vi "Build queue.vi"(8 "Scan settings array":T1[](array[typedef]) {"J-t Illumination conditions" items=["Light only", "Dark only", "Light then dark", "Dark then light"]; "No. of scan rate steps" min=1.0 step=1.0; "Illumination conditions" items=["Light only", "Dark only", "Light then dark", "Dark then light", "Light then dark then light", "Dark then light then dark"]; "Time Constant (s)" items=["0.003", "0.01", "0.03", "0.1", "0.3", "1", "3", "10", "30", "100"]; "Only repeat for best pixel" items=["only for best pixel", "for best 2 pixels", "for best 3 pixels", "for best 4 pixels", "for best 5 pixels", "for best 6 pixels", "for best 7 pixels", "for all pixels"]; "No. of repeat scans" min=1.0 step=1.0; "EQE best pixel only" items=["only the best pixel", "the best 2 pixel", "the best 3 pixel", "the best 4 pixel", "the best 5 pixel", "the best 6 pixel", "the best 7 pixel", "all pixels"]; "P dep best pixel only" items=["only the best pixel", "the best 2 pixels", "the best 3 pixels", "the best 4 pixels", "the best 5 pixels", "the best 6 pixels", "the best 7 pixels", "all pixels"]; "Max power best pixel only" items=["only the best pixel", "the best 2 pixels", "the best 3 pixels", "the best 4 pixels", "the best 5 pixels", "the best 6 pixels", "the best 7 pixels", "all pixels"]; "J-t best pixel only" items=["only the best pixel", "the best 2 pixels", "the best 3 pixels", "the best 4 pixels", "the best 5 pixels", "the best 6 pixels", "the best 7 pixels", "all pixels"]; "Integration time" items=["Fast", "Normal", "High Accuracy"]; "Stabilisation mode" items=["V", "I"]; "Measurement delay (ms)" min=10.0}, 11 "Cell Settings Array":T4(array[cluster])=[{"Cell Position"=1, "Cell Label"="", "Pixel to measure"=0, "Area (cm^2)"=0.126, "Variable"="", "Variable value"="", "Scan settings in queue"=0}, {"Cell Position"=2, "Cell Label"="", "Pixel to measure"=0, "Area (cm^2)"=0.126, "Variable"="", "Variable value"="", "Scan settings in queue"=0}, {"Cell Position"=3, "Cell Label"="", "Pixel to measure"=0, "Area (cm^2)"=0.126, "Variable"="", "Variable value"="", "Scan settings in queue"=0}, {"Cell Position"=4, "Cell Label"="", "Pixel to measure"=0, "Area (cm^2)"=0.126, "Variable"="", "Variable value"="", "Scan settings in queue"=0}, {"Cell Position"=5, "Cell Label"="", "Pixel to measure"=0, "Area (cm^2)"=0.126, "Variable"="", "Variable value"="", "Scan settings in queue"=0}, {"Cell Position"=6, "Cell Label"="", "Pixel to measure"=0, "Area (cm^2)"=0.126, "Variable"="", "Variable value"="", "Scan settings in queue"=0}, {"Cell Position"=7, "Cell Label"="", "Pixel to measure"=0, "Area (cm^2)"=0.126, "Variable"="", "Variable value"="", "Scan settings in queue"=0}, {"Cell Position"=8, "Cell Label"="", "Pixel to measure"=0, "Area (cm^2)"=0.126, "Variable"="", "Variable value"="", "Scan settings in queue"=0}, {"Cell Position"=9, "Cell Label"="", "Pixel to measure"=0, "Area (cm^2)"=0.126, "Variable"="", "Variable value"="", "Scan settings in queue"=0}, {"Cell Position"=10, "Cell Label"="", "Pixel to measure"=0, "Area (cm^2)"=0.126, "Variable"="", "Variable value"="", "Scan settings in queue"=0}, {"Cell Position"=11, "Cell Label"="", "Pixel to measure"=0, "Area (cm^2)"=0.126, "Variable"="", "Variable value"="", "Scan settings in queue"=0}, {"Cell Position"=12, "Cell Label"="", "Pixel to measure"=0, "Area (cm^2)"=0.126, "Variable"="", "Variable value"="", "Scan settings in queue"=0}, {"Cell Position"=13, "Cell Label"="", "Pixel to measure"=0, "Area (cm^2)"=0.126, "Variable"="", "Variable value"="", "Scan settings in queue"=0}, {"Cell Position"=14, "Cell Label"="", "Pixel to measure"=0, "Area (cm^2)"=0.126, "Variable"="", "Variable value"="", "Scan settings in queue"=0}, {"Cell Position"=15, "Cell Label"="", "Pixel to measure"=0, "Area (cm^2)"=0.126, "Variable"="", "Variable value"="", "Scan settings in queue"=0}, {"Cell Position"=16, "Cell Label"="", "Pixel to measure"=0, "Area (cm^2)"=0.126, "Variable"="", "Variable value"="", "Scan settings in queue"=0}] {"Pixel to measure" items=["All", "1", "2", "3", "4", "5", "6", "7", "8"]}) -> (3 "Measurement queue":T3(array[cluster]) {"Pixel to measure" items=["All", "1", "2", "3", "4", "5", "6", "7", "8"]})   [LabVIEW 2011]
uses:
  TypeDefs/Scan settings.ctl
  TypeDefs/Settings Boolean.ctl
panel:
  out "Max power best pixel only":u16
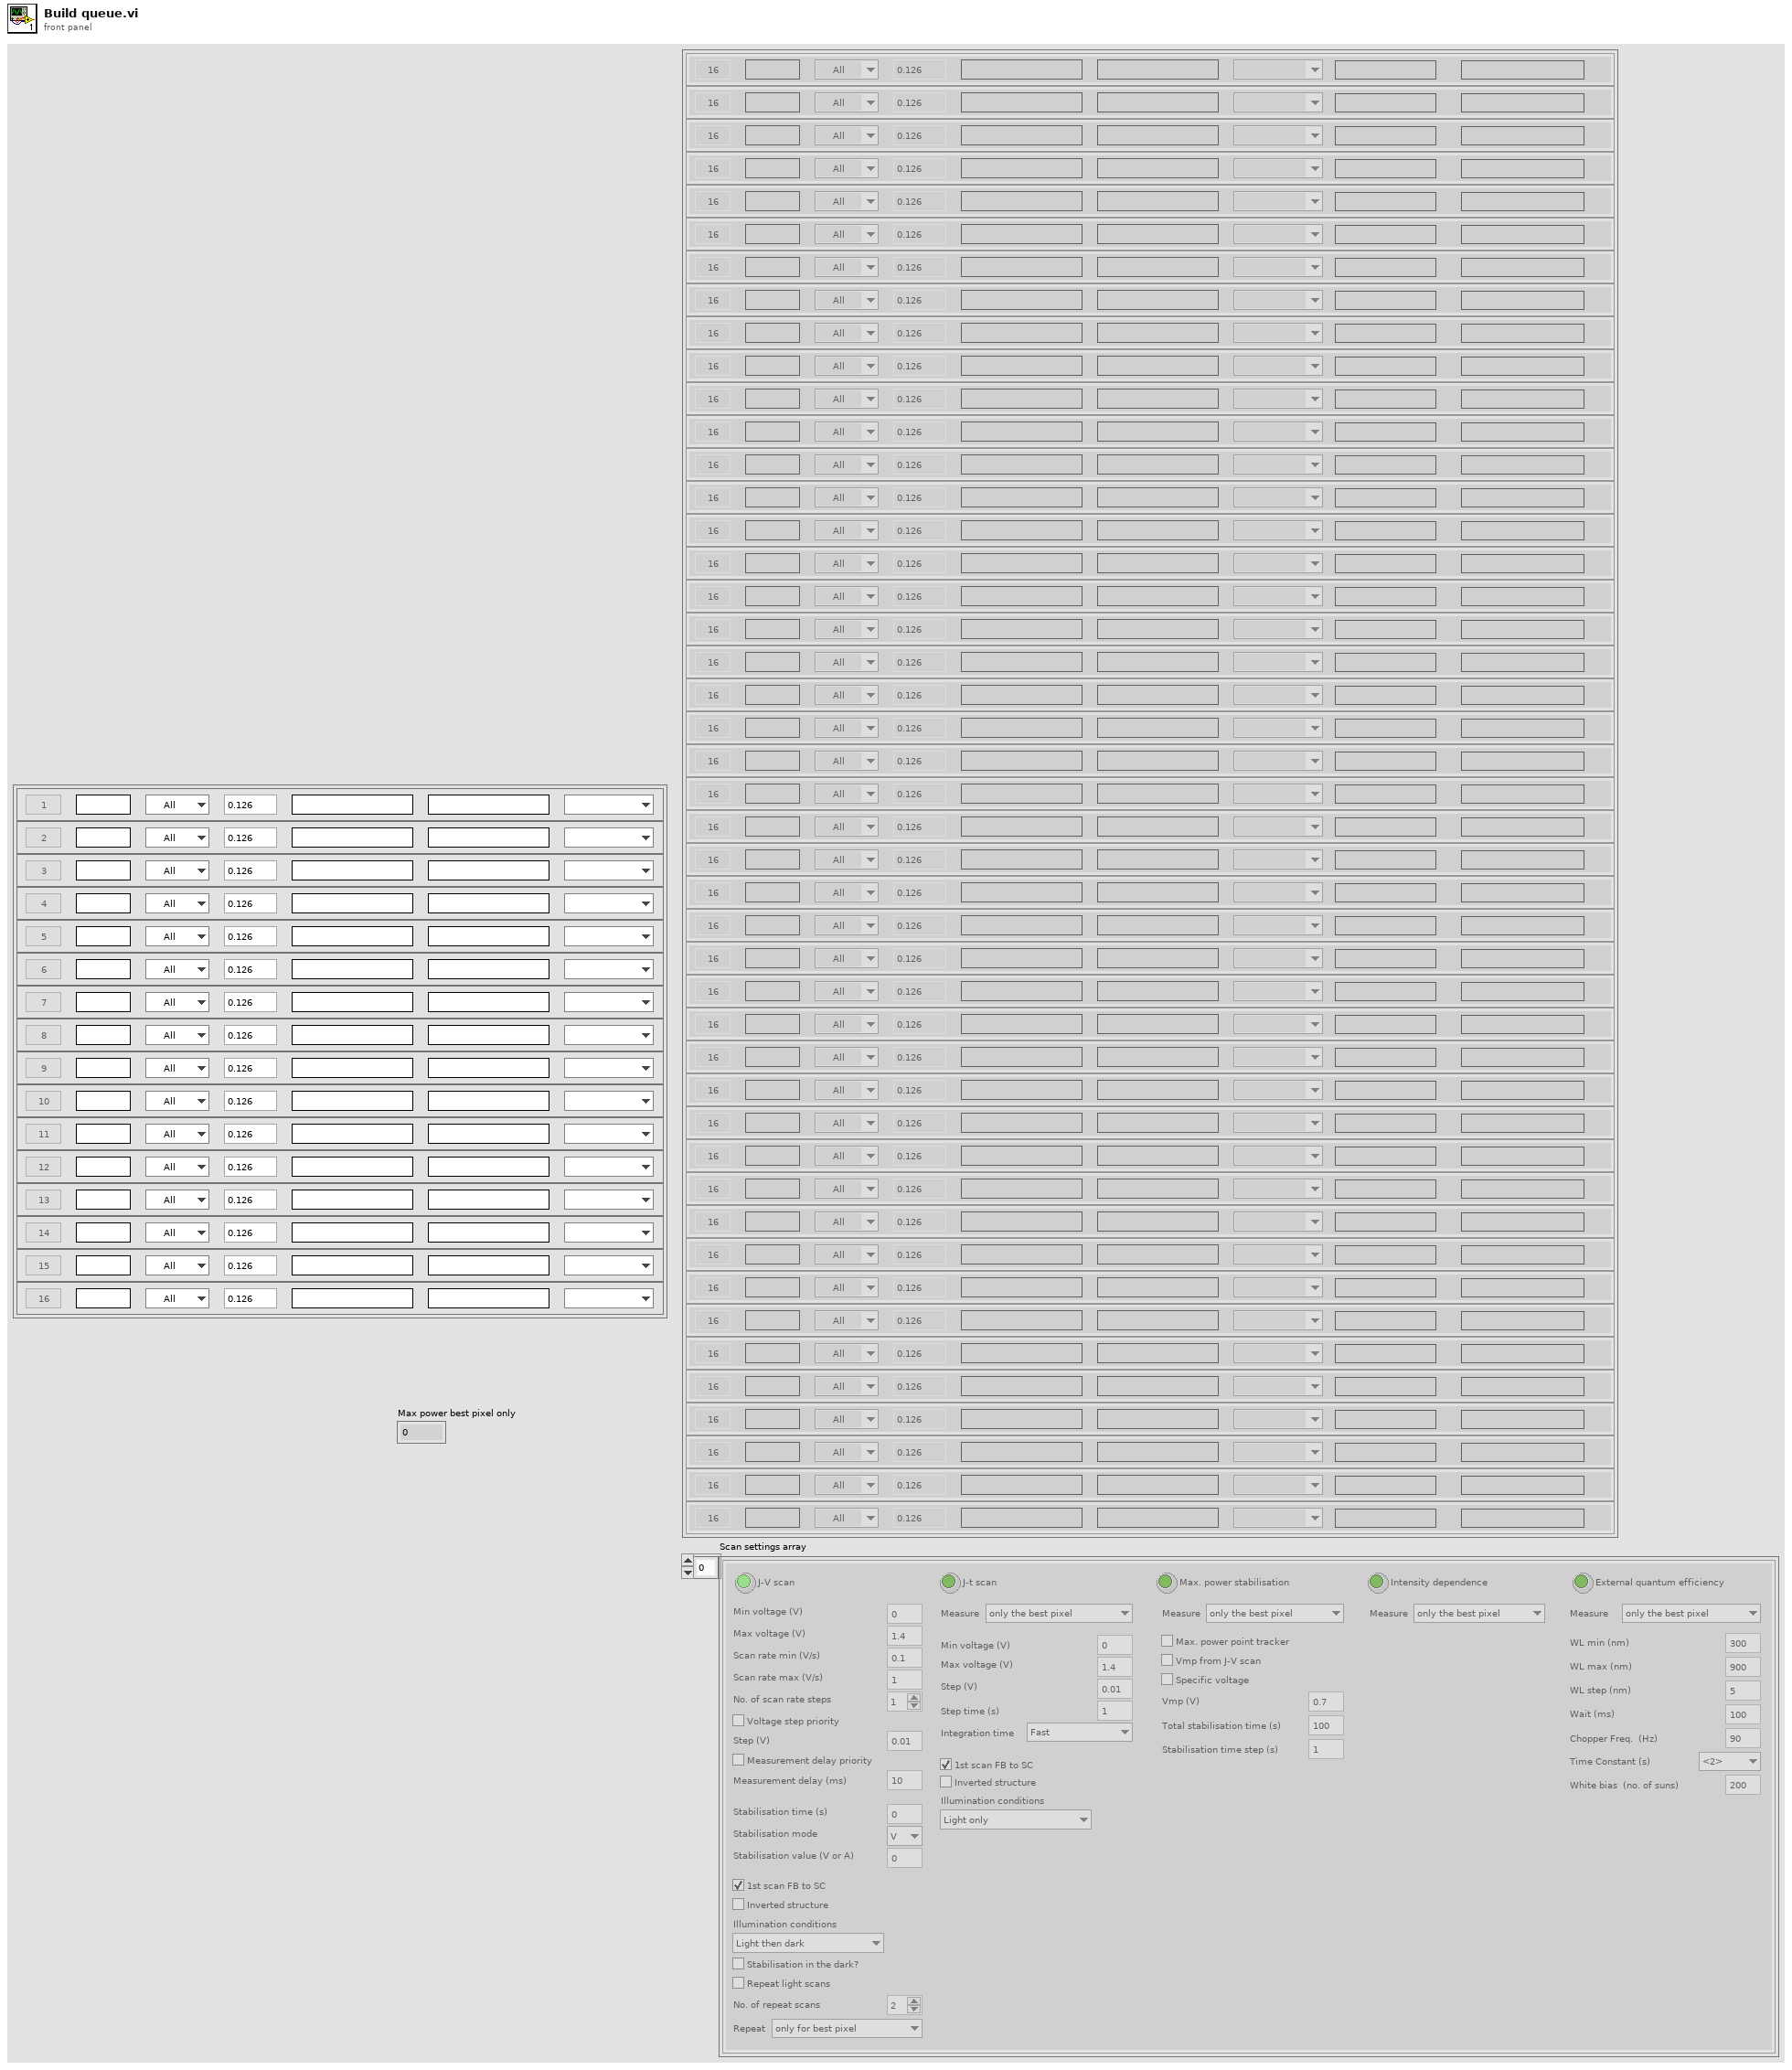
[diagram p1: front panel]
types:
  T1 = typedef "Scan settings.ctl" = cluster{"J-V scan":T2, "J-t scan":bool, "Min voltage (V)":dbl, "Max voltage (V)":dbl, "Step (V)":dbl, "Measurement delay (ms)":dbl, "1st scan FB-SC":bool, "Inverted structure":bool, "Stabilisation time (s)":dbl, "Stabilisation mode":u16, "Stabilisation value (V or A) ":dbl, "Step time (s)":dbl, "Integration time":u16, "Repeat light scans":bool, "Stabilisation in the dark?":bool, "J-t Min (V)":dbl, "J-t Max (V)":dbl, "J-t Step (V)":dbl, "Max. power stabilisation":bool, "J-t 1st scan FB-SC":bool, "J-t Inverted structure":bool, "Max power tracking":bool, "Vmp (V)":dbl, "Total stabilisation time (s)":dbl, "J-t best pixel only":u16, "Max power best pixel only":u16, "Vmp from J-V scan":bool, "Intensity dependence":bool, "P dep best pixel only":u16, "External quantum efficiency":bool, "EQE best pixel only":u16, "WL min (nm)":dbl, "WL max (nm)":dbl, "WL step (nm)":dbl, "Wait (ms)":dbl, "No. of repeat scans":dbl, "Only repeat for best pixel":u16, "Chopper Freq.  (Hz)":dbl, "Time Constant (s)":dbl, "Stabilisation time step (s)":dbl, "Illumination conditions":u16, "Scan rate min (V/s)":dbl, "Scan rate max (V/s)":dbl, "No. of scan rate steps":dbl, "Scan rate voltage step priority":bool, "Scan rate measurement delay priority":bool, "J-t Illumination conditions":u16, "White bias  (no. of suns)":dbl, "Max P stab. Specific voltage":bool}
  T2 = typedef "Settings Boolean.ctl" = bool
  T3 = cluster{"Cell Position":i32, "Cell Label":string, "Pixel to measure":u16, "Area (cm^2)":dbl, "Variable":string, "Variable value":string, "Scan settings in queue":u16, "Light or dark":string, "Measurement type":string}[]
  T4 = cluster{"Cell Position":i32, "Cell Label":string, "Pixel to measure":u16, "Area (cm^2)":dbl, "Variable":string, "Variable value":string, "Scan settings in queue":u16}[]
  T5 = cluster{"Cell Position":i32, "Cell Label":string, "Pixel to measure":u16, "Area (cm^2)":dbl, "Variable":string, "Variable value":string, "Scan settings in queue":u16}
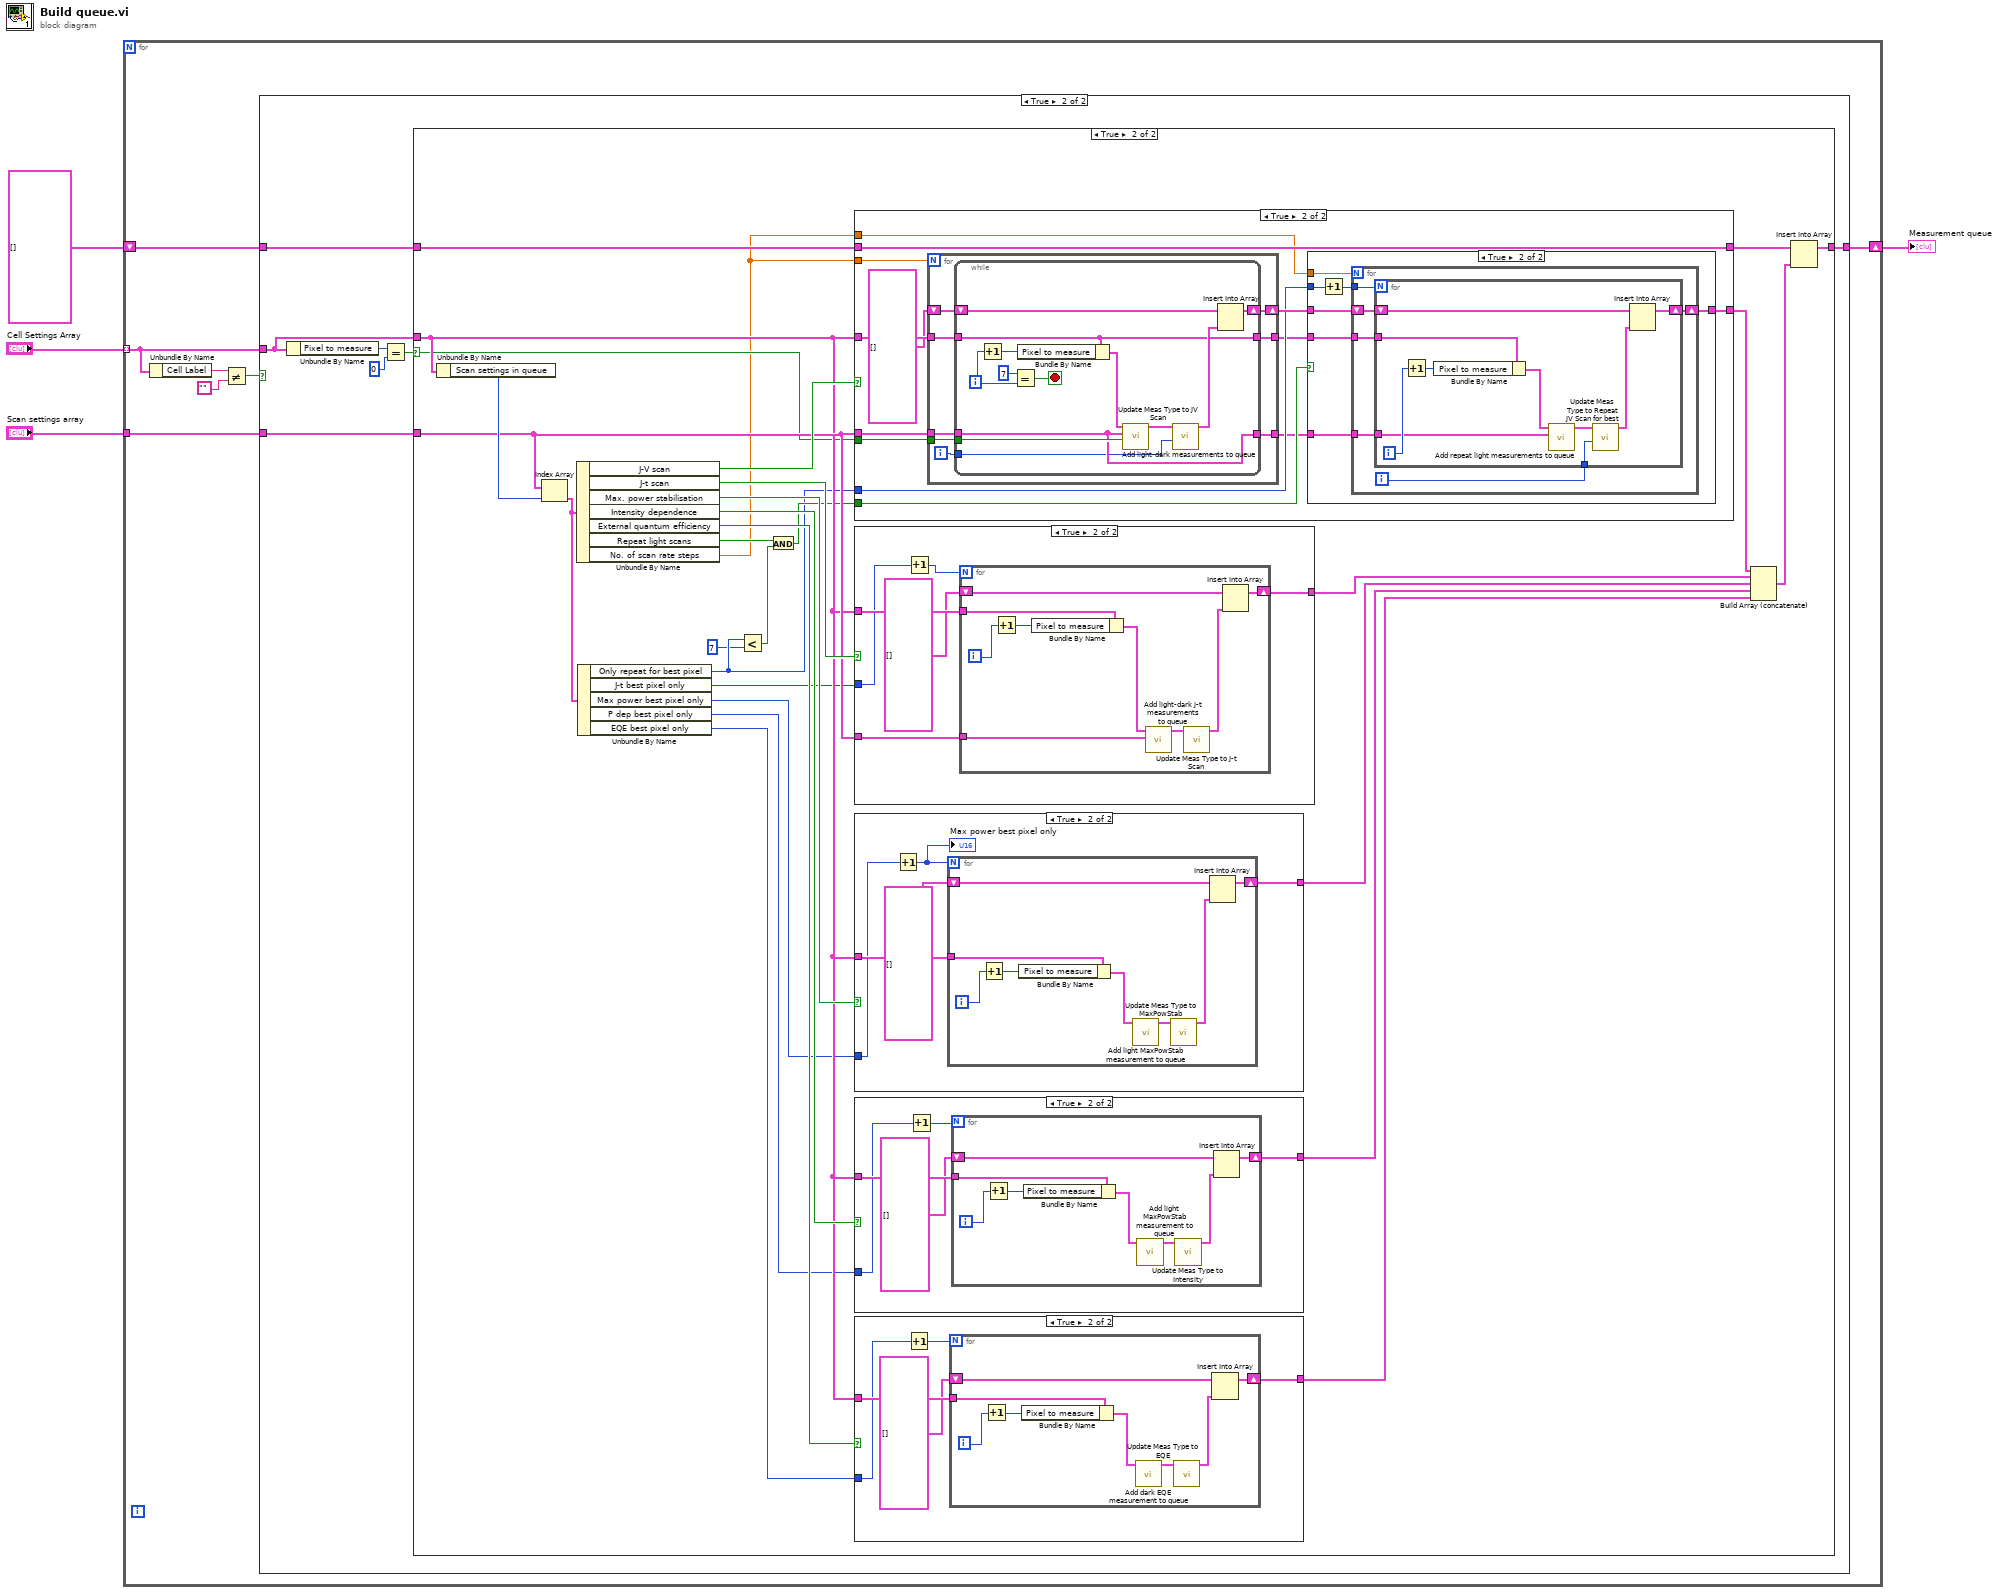
[diagram p0: block diagram]
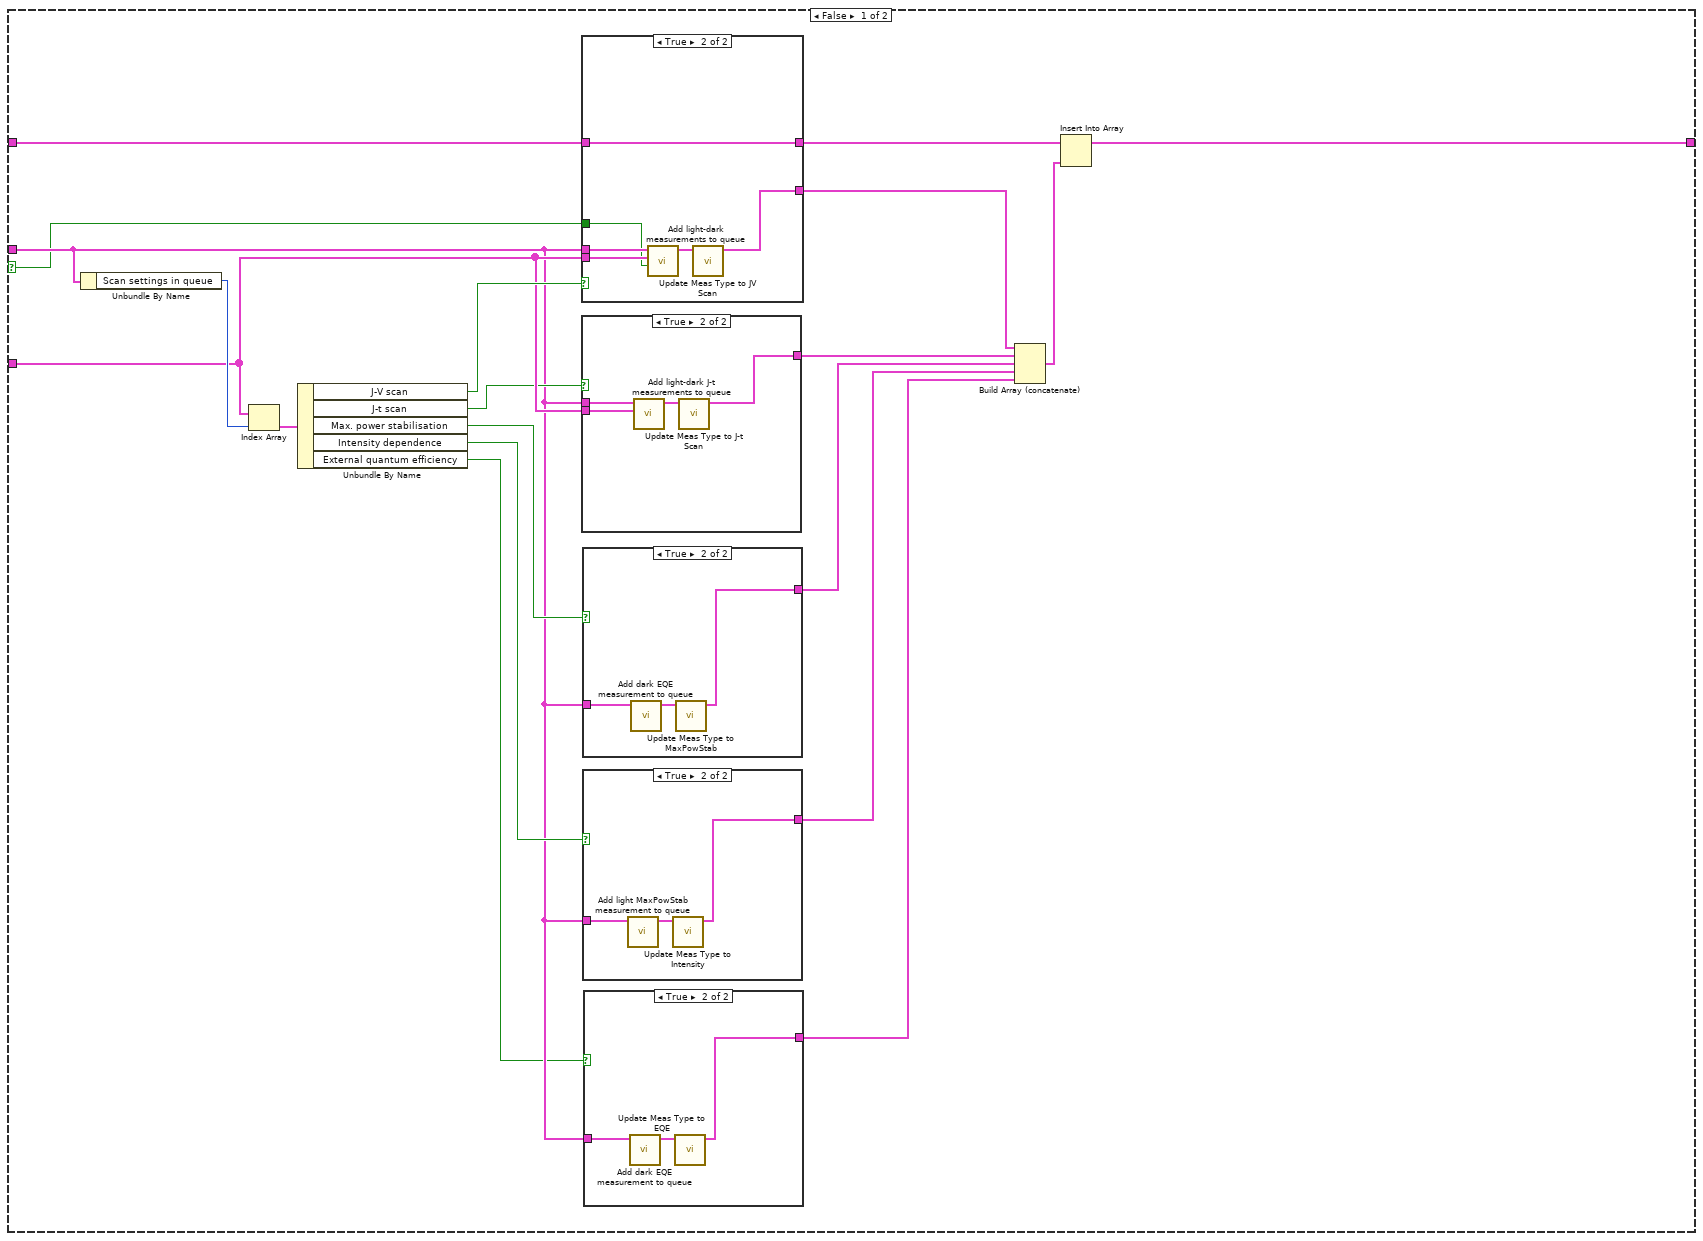
[diagram p3: hidden frame]
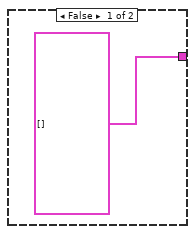
[diagram p4: hidden frame]
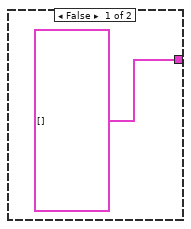
[diagram p5: hidden frame]
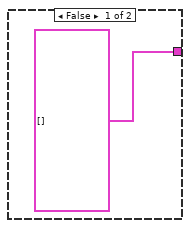
[diagram p6: hidden frame]
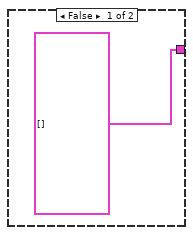
[diagram p7: hidden frame]
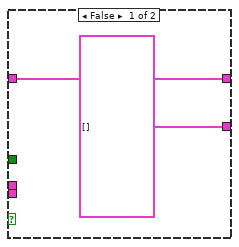
[diagram p8: hidden frame]
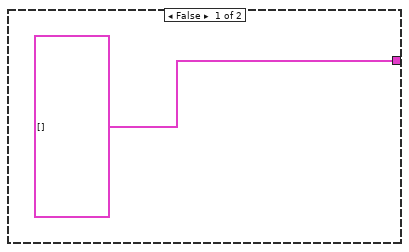
[diagram p9: hidden frame]
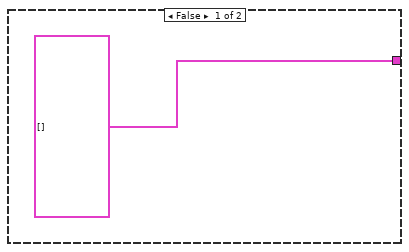
[diagram p10: hidden frame]
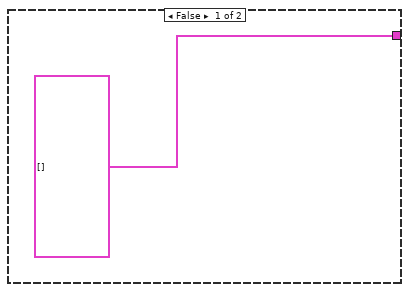
[diagram p11: hidden frame]
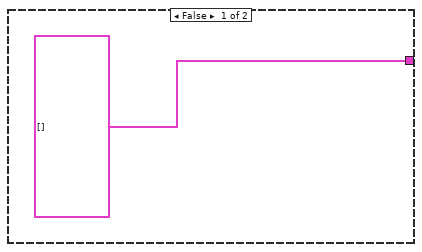
[diagram p12: hidden frame]
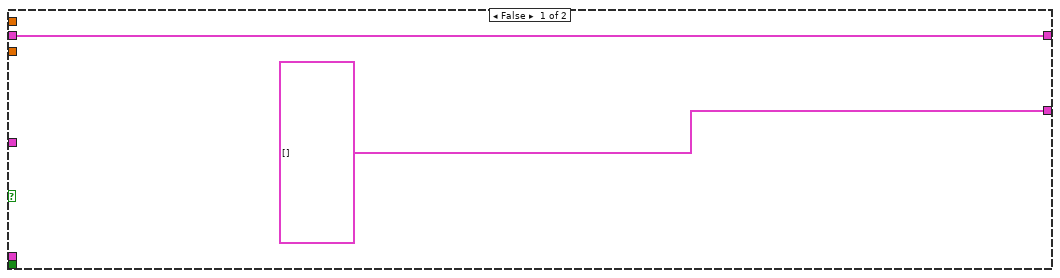
[diagram p13: hidden frame]
diagram:
  n1 = for {
    tunnel: "Cell Settings Array" -> [w10] mode=indexing
    shift-right: [w11] -> w2
    shift-left: T3 [] ("Measurement queue") -> [w6]
    tunnel: "Scan settings array" -> [w5]
    n2 = Unbundle By Name(w10) -> ("Cell Label"=w9:string)
    n3 = Not Equal?(x=w9, y="") -> (x != y?=w7:bool)
    n4 = case shown="True" w7 {
      tunnel: [w12 w16] -> w11
      tunnel: w10 -> [_ w15]
      tunnel: w6 -> [w12 w14]
      tunnel: w5 -> [_ w13]
      frame False {
      }
      frame True {
        n5 = Unbundle By Name(w15) -> ("Pixel to measure"=w19:u16)
        n6 = Equal?(x=w19, y=0) -> (x = y?=w17:bool)
        n7 = case shown="True" w17 {
          selector: w17 -> [w20 w70]
          tunnel: w15 -> [w24 w81]
          tunnel: [w38 w90] -> w16
          tunnel: w14 -> [w25 w80]
          tunnel: w13 -> [w34 w86]
          frame False {
            n8 = Unbundle By Name(w24) -> ("Scan settings in queue"=w37:u16)
            n9 = Index Array(array=w34, index=w37) -> (element=w22:T1)
            n10 = Unbundle By Name(w22) -> ("J-V scan"=w35:T2, "J-t scan"=w33:bool, "Max. power stabilisation"=w27:bool, "Intensity dependence"=w26:bool, "External quantum efficiency"=w23:bool)
            n11 = case shown="True" w35 {
              tunnel: w24 -> [_ w62]
              tunnel: w34 -> [_ w61]
              tunnel: [w57 w60] -> w36
              tunnel: w25 -> [w57 w60]
              tunnel: [T3 [] ("Measurement queue") w59] -> w21
              tunnel: w20 -> [_ w58]
              frame False {
              }
              frame True {
                n12 = call "Add light-dark measurements to queue.vi"("Measuring all pixels on cell?"=w58, "Scan settings array"=w61, "Cell settings cluster"=w62) -> ("Light/dark array"=w63:T3)  [unwired: 8 in]
                n13 = call "Update Meas Type to JV Scan.vi"("Cell details array in"=w63) -> ("Cell details array out"=w59:T3)  [unwired: 10 in]
              }
            }
            n14 = case shown="True" w33 {
              tunnel: w24 -> [_ w54]
              tunnel: w34 -> [_ w53]
              tunnel: [T3 [] ("Measurement queue") w52] -> w32
              frame False {
              }
              frame True {
                n15 = call "Add light-dark J-t measurements to queue.vi"("Scan settings array"=w53, "Cell settings cluster"=w54) -> ("Light/dark array"=w55:T3)  [unwired: 9 in]
                n16 = call "Update Meas Type to J-t Scan.vi"("Cell details array in"=w55) -> ("Cell details array out"=w52:T3)  [unwired: 10 in]
              }
            }
            n17 = case shown="True" w27 {
              tunnel: [T3 [] ("Measurement queue") w48] -> w31
              tunnel: w24 -> [_ w49]
              frame False {
              }
              frame True {
                n18 = call "Add dark EQE measurement to queue.vi"("Cell settings cluster"=w49) -> ("Light/dark array"=w50:T3)  [unwired: 10 in]
                n19 = call "Update Meas Type to MaxPowStab.vi"("Cell details array in"=w50) -> ("Cell details array out"=w48:T3)  [unwired: 10 in]
              }
            }
            n20 = case shown="True" w26 {
              tunnel: [T3 [] ("Measurement queue") w44] -> w30
              tunnel: w24 -> [_ w45]
              frame False {
              }
              frame True {
                n21 = call "Add light MaxPowStab measurement to queue.vi"("Cell settings cluster"=w45) -> ("Light/dark array"=w46:T3)  [unwired: 10 in]
                n22 = call "Update Meas Type to Intensity.vi"("Cell details array in"=w46) -> ("Cell details array out"=w44:T3)  [unwired: 10 in]
              }
            }
            n23 = case shown="True" w23 {
              tunnel: [T3 [] ("Measurement queue") w40] -> w29
              tunnel: w24 -> [_ w41]
              frame False {
              }
              frame True {
                n24 = call "Add dark EQE measurement to queue.vi"("Cell settings cluster"=w41) -> ("Light/dark array"=w42:T3)  [unwired: 10 in]
                n25 = call "Update Meas Type to EQE.vi"("Cell details array in"=w42) -> ("Cell details array out"=w40:T3)  [unwired: 10 in]
              }
            }
            n26 = Build Array (concatenate)(w21, w32, w31, w30, w29) -> (w28:T3)
            n27 = Insert Into Array(array=w36, new element=w28) -> (w38:T3)  [unwired: 1 in]
          }
          frame True {
            n28 = Unbundle By Name(w81) -> ("Scan settings in queue"=w92:u16)
            n29 = Index Array(array=w86, index=w92) -> (element=w75:T1)
            n30 = Unbundle By Name(w75) -> ("J-V scan"=w91:T2, "J-t scan"=w87:bool, "Max. power stabilisation"=w85:bool, "Intensity dependence"=w83:bool, "External quantum efficiency"=w79:bool, "Repeat light scans"=w69:bool, "No. of scan rate steps"=w66:dbl)
            n31 = Unbundle By Name(w75) -> ("Only repeat for best pixel"=w65:u16, "J-t best pixel only"=w74:u16, "Max power best pixel only"=w73:u16, "P dep best pixel only"=w72:u16, "EQE best pixel only"=w71:u16)
            n32 = Less?(x=w65, y=u16 7 ("x")) -> (x < y?=w68:bool)
            n33 = And(x=w69, y=w68) -> (x .and. y?=w67:bool)
            n34 = case shown="True" w91 {
              tunnel: [w152 w163] -> w77
              tunnel: w80 -> [w152 w163]
              tunnel: w81 -> [_ w165]
              tunnel: w86 -> [_ w164]
              tunnel: [T3 [] ("Measurement queue") w161] -> w76
              tunnel: w70 -> [_ w162]
              tunnel: w67 -> [_ w159]
              tunnel: w65 -> [_ w158]
              tunnel: w66 -> [_ w155]
              tunnel: w66 -> [_ w153]
              frame False {
              }
              frame True {
                n35 = for {
                  N: w155 -> [_]
                  tunnel: w165 -> [w173]
                  tunnel: w164 -> [w172]
                  tunnel: w162 -> [w171]
                  tunnel: [w169] -> w157
                  tunnel: [w168] -> w156
                  shift-right: [w170] -> w160
                  shift-left: T3 [] ("Measurement queue") -> [w166]
                  i -> [w167]
                  n36 = while {
                    tunnel: w173 -> [w176]
                    shift-right: [w182] -> w170
                    shift-left: w166 -> [w181]
                    tunnel: w172 -> [w175]
                    tunnel: w171 -> [w177]
                    tunnel: [w176] -> w169
                    tunnel: [w175] -> w168
                    tunnel: w167 -> [w174]
                    i -> [w184]
                    stop <- w186 stop-if-true
                    n37 = Increment(x=w184) -> (x+1=w185:i32)
                    n38 = Equal?(x=7, y=w184) -> (x = y?=w186:bool)
                    n39 = Bundle By Name(cluster=w176, "Pixel to measure"=w185) -> (w180:T5)
                    n40 = call "Add light-dark measurements to queue.vi"("Measuring all pixels on cell?"=w177, "Scan settings array"=w175, "Cell settings cluster"=w180) -> ("Light/dark array"=w179:T3)  [unwired: 8 in]
                    n41 = call "Update Meas Type to JV Scan.vi"("Scan rate step number"=w174, "Cell details array in"=w179) -> ("Cell details array out"=w178:T3)  [unwired: 9 in]
                    n42 = Insert Into Array(array=w181, new element=w178) -> (w182:T3)  [unwired: 1 in]
                  }
                }
                n43 = case shown="True" w159 {
                  tunnel: [w187 w193] -> w161
                  tunnel: w160 -> [w187 w194]
                  tunnel: w158 -> [_ w189]
                  tunnel: w157 -> [_ w192]
                  tunnel: w156 -> [_ w191]
                  tunnel: w153 -> [_ w190]
                  frame False {
                  }
                  frame True {
                    n44 = Increment(x=w189) -> (x+1=w188:u16)
                    n45 = for {
                      N: w190 -> [_]
                      tunnel: w188 -> [w198]
                      tunnel: w192 -> [w197]
                      tunnel: w191 -> [w196]
                      shift-right: [w199] -> w193
                      shift-left: w194 -> [w200]
                      i -> [w195]
                      n46 = for {
                        N: w198 -> [_]
                        shift-right: [w209] -> w199
                        shift-left: w200 -> [w210]
                        tunnel: w197 -> [w204]
                        tunnel: w196 -> [w203]
                        tunnel: w195 -> [w201]
                        i -> [w208]
                        n47 = Increment(x=w208) -> (x+1=w207:i32)
                        n48 = Bundle By Name(cluster=w204, "Pixel to measure"=w207) -> (w206:T5)
                        n49 = call "Add repeat light measurements to queue.vi"("Scan settings array"=w203, "Cell settings cluster"=w206) -> ("Repeat light array"=w205:T3)  [unwired: 9 in]
                        n50 = call "Update Meas Type to Repeat JV Scan for best.vi"("Scan rate step number"=w201, "Cell details array in"=w205) -> ("Cell details array out"=w202:T3)  [unwired: 9 in]
                        n51 = Insert Into Array(array=w210, new element=w202) -> (w209:T3)  [unwired: 1 in]
                      }
                    }
                  }
                }
              }
            }
            n52 = case shown="True" w87 {
              tunnel: [T3 [] ("Measurement queue") w141] -> w88
              tunnel: w81 -> [_ w140]
              tunnel: w86 -> [_ w139]
              tunnel: w74 -> [_ w136]
              frame False {
              }
              frame True {
                n53 = Increment(x=w136) -> (x+1=w137:u16)
                n54 = for {
                  N: w137 -> [_]
                  tunnel: w140 -> [w148]
                  shift-right: [w147] -> w141
                  shift-left: T3 [] ("Measurement queue") -> [w146]
                  tunnel: w139 -> [w144]
                  i -> [w149]
                  n55 = Increment(x=w149) -> (x+1=w150:i32)
                  n56 = Bundle By Name(cluster=w148, "Pixel to measure"=w150) -> (w145:T5)
                  n57 = call "Add light-dark J-t measurements to queue.vi"("Scan settings array"=w144, "Cell settings cluster"=w145) -> ("Light/dark array"=w143:T3)  [unwired: 9 in]
                  n58 = call "Update Meas Type to J-t Scan.vi"("Cell details array in"=w143) -> ("Cell details array out"=w142:T3)  [unwired: 10 in]
                  n59 = Insert Into Array(array=w146, new element=w142) -> (w147:T3)  [unwired: 1 in]
                }
              }
            }
            n60 = case shown="True" w85 {
              tunnel: [T3 [] ("Measurement queue") w126] -> w84
              tunnel: w81 -> [_ w125]
              tunnel: w73 -> [_ w123]
              frame False {
              }
              frame True {
                n61 = Increment(x=w123) -> (x+1=w122:u16)
                "Max power best pixel only" <- w122
                n62 = for {
                  N: w122 -> [_]
                  tunnel: w125 -> [w132]
                  shift-right: [w131] -> w126
                  shift-left: T3 [] ("Measurement queue") -> [w130]
                  i -> [w133]
                  n63 = Increment(x=w133) -> (x+1=w134:i32)
                  n64 = Bundle By Name(cluster=w132, "Pixel to measure"=w134) -> (w129:T5)
                  n65 = call "Add light MaxPowStab measurement to queue.vi"("Cell settings cluster"=w129) -> ("Light/dark array"=w128:T3)  [unwired: 10 in]
                  n66 = call "Update Meas Type to MaxPowStab.vi"("Cell details array in"=w128) -> ("Cell details array out"=w127:T3)  [unwired: 10 in]
                  n67 = Insert Into Array(array=w130, new element=w127) -> (w131:T3)  [unwired: 1 in]
                }
              }
            }
            n68 = case shown="True" w83 {
              tunnel: [T3 [] ("Measurement queue") w112] -> w82
              tunnel: w81 -> [_ w111]
              tunnel: w72 -> [_ w108]
              frame False {
              }
              frame True {
                n69 = Increment(x=w108) -> (x+1=w109:u16)
                n70 = for {
                  N: w109 -> [_]
                  tunnel: w111 -> [w118]
                  shift-right: [w117] -> w112
                  shift-left: T3 [] ("Measurement queue") -> [w116]
                  i -> [w119]
                  n71 = Increment(x=w119) -> (x+1=w120:i32)
                  n72 = Bundle By Name(cluster=w118, "Pixel to measure"=w120) -> (w115:T5)
                  n73 = call "Add light MaxPowStab measurement to queue.vi"("Cell settings cluster"=w115) -> ("Light/dark array"=w114:T3)  [unwired: 10 in]
                  n74 = call "Update Meas Type to Intensity.vi"("Cell details array in"=w114) -> ("Cell details array out"=w113:T3)  [unwired: 10 in]
                  n75 = Insert Into Array(array=w116, new element=w113) -> (w117:T3)  [unwired: 1 in]
                }
              }
            }
            n76 = case shown="True" w79 {
              tunnel: [T3 [] ("Measurement queue") w98] -> w78
              tunnel: w81 -> [_ w97]
              tunnel: w71 -> [_ w94]
              frame False {
              }
              frame True {
                n77 = Increment(x=w94) -> (x+1=w95:u16)
                n78 = for {
                  N: w95 -> [_]
                  tunnel: w97 -> [w104]
                  shift-right: [w103] -> w98
                  shift-left: T3 [] ("Measurement queue") -> [w102]
                  i -> [w105]
                  n79 = Increment(x=w105) -> (x+1=w106:i32)
                  n80 = Bundle By Name(cluster=w104, "Pixel to measure"=w106) -> (w101:T5)
                  n81 = call "Add dark EQE measurement to queue.vi"("Cell settings cluster"=w101) -> ("Light/dark array"=w100:T3)  [unwired: 10 in]
                  n82 = call "Update Meas Type to EQE.vi"("Cell details array in"=w100) -> ("Cell details array out"=w99:T3)  [unwired: 10 in]
                  n83 = Insert Into Array(array=w102, new element=w99) -> (w103:T3)  [unwired: 1 in]
                }
              }
            }
            n84 = Build Array (concatenate)(w76, w88, w84, w82, w78) -> (w89:T3)
            n85 = Insert Into Array(array=w77, new element=w89) -> (w90:T3)  [unwired: 1 in]
          }
        }
      }
    }
  }
  "Measurement queue" <- w2
